vi "swerveAuto.vi"(3 "heading (360)":dbl, 4 "direction (360)":dbl, 5 "distance (units)":dbl) -> (0 "section complete":bool, 1 "drivePower":dbl[](array[numeric]), 2 "steerPower":dbl[](array[numeric]))   [LabVIEW 2019]
uses:
  swerveData.vi
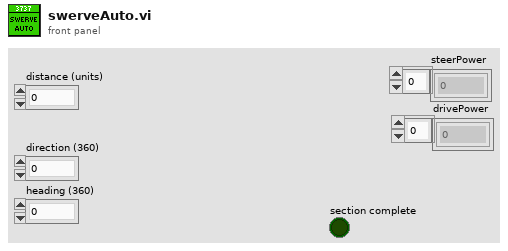
[diagram p1: front panel]
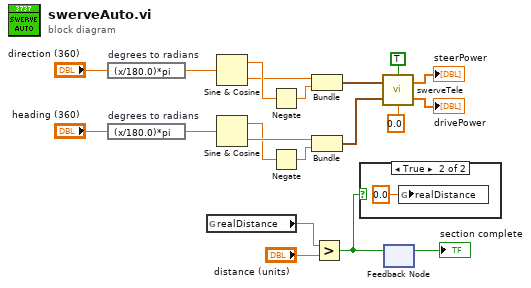
[diagram p0: block diagram]
diagram:
  n1 = expression code="(x/180.0)*pi" "degrees to radians"("direction (360)") -> (w19:dbl)
  n2 = expression code="(x/180.0)*pi" "degrees to radians"("heading (360)") -> (w18:dbl)
  n3 = global read "swerveData.vi" "realDistance"() -> (w15:dbl)
  n4 = Sine & Cosine(0:w19) -> (1:w4:dbl, 2:w3:dbl)
  n5 = Sine & Cosine(0:w18) -> (1:w6:dbl, 2:w7:dbl)
  n6 = Negate(x=w4) -> (-x=w5:dbl)
  n7 = Negate(x=w6) -> (-x=w10:dbl)
  n8 = Bundle(w3, w5) -> (w2:cluster{dbl, dbl})  [unwired: 1 in]
  n9 = Bundle(w7, w10) -> (w1:cluster{dbl, dbl})  [unwired: 1 in]
  n10 = Greater?(x=w15, y="distance (units)") -> (0:w9:bool)
  n11 = case shown="True" w9 {
    frame False {
    }
    frame True {
      n12 = global write "swerveData.vi" "realDistance"(0.0 ("realDistance")) -> ()
    }
  }
  n13 = call "swerveTele.vi"("joystickRight(x,y)"=w1, "rotation"=0.0, "joystickLeft(x,y)"=w2, "feildCentric"=TRUE) -> ("drivePower"=→"drivePower":dbl[], "steerPower"=→"steerPower":dbl[])
  n14 = feedback-in #1(w9) -> ()
  n15 = feedback #1() -> (→"section complete":bool)  [unwired: 1 in]
